vi "AT Get Enum String By Index A.vi"(8 "error in (no error)":errorcluster, 9 "Index":i32, 10 "Feature":string, 11 "Handle":i32) -> (0 "error out":errorcluster, 2 "String":string, 3 "Status":i32)   [LabVIEW 2019]
doc: "GetEnumStringByIndex\n\nOutput:\n I32 Status\n String Value\n\nInput:\n I32 Handle\n String Feature\n I32 Value\n\nThis function returns the text representation of the specified enumerated feature index. The index should be in the range 0... Count-1, where Count has been retrieved using the AT_GetEnumCount function."
uses:
  atcoreA.dll
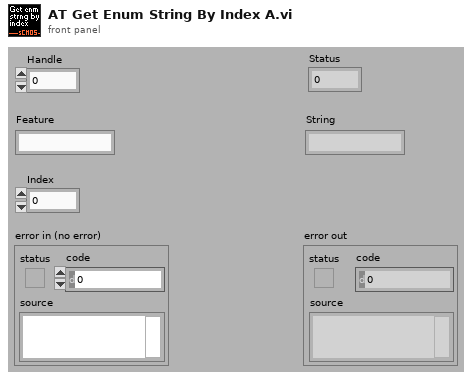
[diagram p1: front panel]
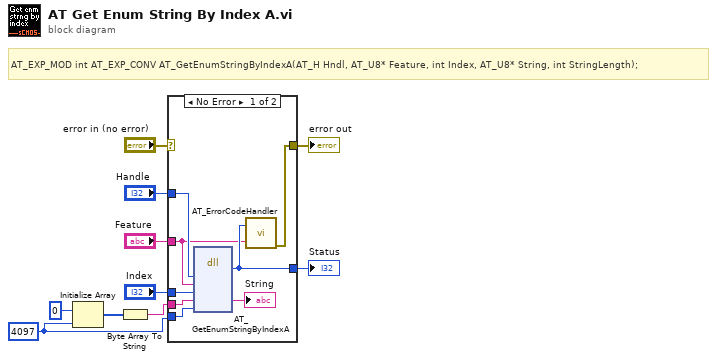
[diagram p0: block diagram]
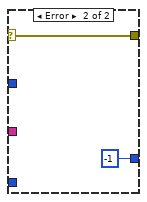
[diagram p2: hidden frame]
diagram:
  w3 = 4097 ("dimension size")
  # "AT_EXP_MOD int AT_EXP_CONV AT_GetEnumStringByIndexA(AT_H Hndl, AT_U8* Feature, int Index, AT_U8* String, int StringLength);"
  n1 = Initialize Array(u8 0 ("element"), w3) -> (w6:u8[])
  n2 = Byte Array To String(unsigned byte array=w6) -> (string=w5:string)
  n3 = case shown="No Error" "error in (no error)" {
    selector: "error in (no error)" -> [_ w20]
    tunnel: [w12 -1] -> w10
    tunnel: "Handle" -> [w18 _]
    tunnel: "Feature" -> [w11 _]
    tunnel: "Index" -> [w17 _]
    tunnel: w5 -> [w16 _]
    tunnel: w3 -> [w14 _]
    tunnel: [w13 w20] -> w1
    frame No Error {
      n4 = dll-call lib="atcoreA.dll" fn="AT_GetEnumStringByIndexA"("Handle"=w18, "Feature"=w11, "Index"=w17, "String"=w16, "StringLength"=w14) -> ("Status"=w12:i32, "String"=→"String":string)  [unwired: 7 in, 2 out]
      n5 = call <userlib>:"AT_ErrorCodeHandler.vi"("Error"=w12, "Feature Name"=w11) -> ("error out"=w13:errorcluster)  [unwired: 5 in]
    }
    frame Error {
    }
  }
  "Status" <- w10
  "error out" <- w1
